vi "p'.vi"() -> ()   [LabVIEW 2013]
panel:
  out "p'":dbl
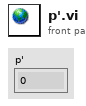
[diagram p1: front panel]
diagram:
